vi "set_samples_to_read.vi"(8 "error in (no error)":errorcluster, 10 "samples to read":i64, 11 "GenericDAQ.lvclass in":refnum<class "GenericDAQ.lvclass">) -> (0 "error out":errorcluster, 3 "GenericDAQ.lvclass out":refnum<class "GenericDAQ.lvclass">)   [LabVIEW 2010, in "GenericDAQ.lvclass"]
uses:
  GenericDAQ.lvclass
  GenericDAQ.lvclass/GenericDAQ.ctl
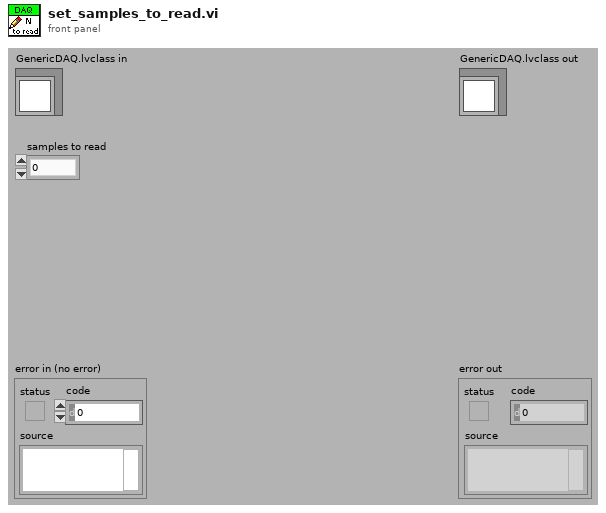
[diagram p1: front panel]
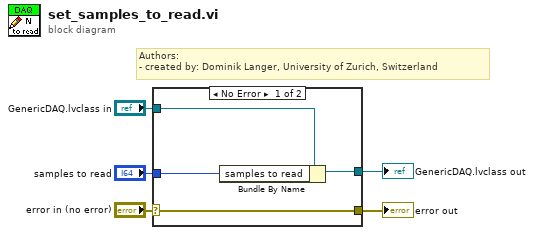
[diagram p0: block diagram]
diagram:
  # "Authors: \n- created by: Dominik Langer, University of Zurich, Switzerland"
  n1 = case shown="No Error" "error in (no error)" {
    selector: "error in (no error)" -> [w9 w10]
    tunnel: [w9 w10] -> w4
    tunnel: [w7 w11] -> w2
    tunnel: "GenericDAQ.lvclass in" -> [w8 w11]
    tunnel: "samples to read" -> [w6 _]
    frame No Error {
      n2 = Bundle By Name(cluster=w8, "samples to read"=w6) -> (w7:refnum<class "GenericDAQ.lvclass">)
    }
    frame Error {
    }
  }
  "error out" <- w4
  "GenericDAQ.lvclass out" <- w2
